vi "Power Accuracy Format Plot.vi"(6 "Calculated Values":refnum<vi>, 8 "error in (no error)":errorcluster, 9 "Reset Plot? (F)":bool, 10 "Test Parameters":T1={"Stimulus"={"Power Start"=38, "Power Stop"=46, "Frequency Type"=enum."Band Edges", "Frequency Points"=[], "TX 1 Frequency (MHz)"={"Min"=0.0, "Max"=0.0}, "TX 2 Frequency (MHz)"={"Min"=0.0, "Max"=0.0}, "RX Frequency (MHz)"={"Min"=0.0, "Max"=0.0}, "Pad Model Number"="", "Pad Serial Number"="", "Pad Values"=[]}, "Measurement"={"DUT Port"=enum."Port 1", "Direction"=0}, "Display"={"Power"={"Min"=0, "Max"=0}, "Tolerance"={"Min"=0.0, "Max"=0.0}}, "Limit"={"Tolerance"=0.35}, "Calibration"={"Calibrated?"=FALSE}} {"Measurement"."Direction" items=["Reverse", "Forward", "Auxiliary"]}, 11 "Plots":T9) -> (0 "error out":errorcluster)   [LabVIEW 2011]
uses:
  TypeDefs/Power Accuracy Test Parameters.ctl
  TypeDefs/Power Accuracy Stimulus Parameters.ctl
  TypeDefs/Power Accuracy Measurement Parameters.ctl
  SI.LIB/PIM.LIB/HW IO/DUTport.ctl
  SI.LIB/PIM.LIB/HW IO/MeasMode.ctl
  TypeDefs/Power Accuracy Display Parameters.ctl
  TypeDefs/Power Accuracy Limit Parameters.ctl
  TypeDefs/Power Accuracy Calibration State.ctl
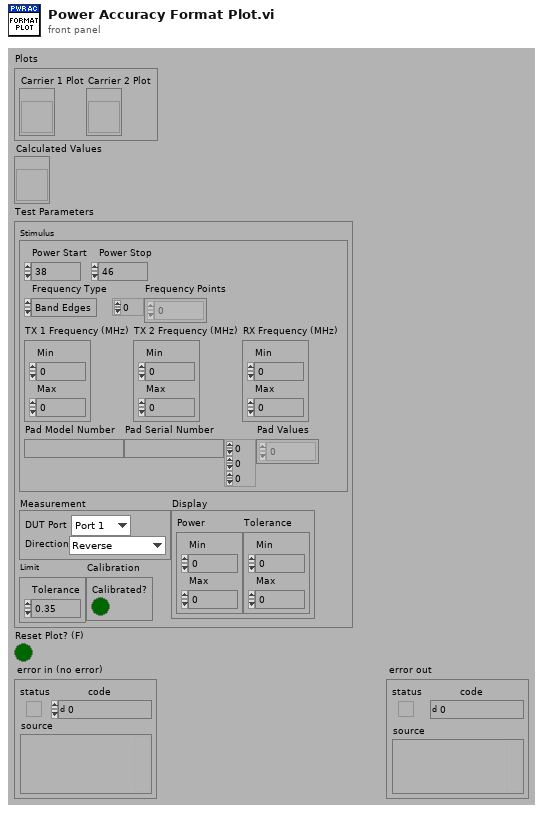
[diagram p1: front panel]
types:
  T1 = typedef "Power Accuracy Test Parameters.ctl" = cluster{"Stimulus":T2, "Measurement":T3, "Display":T6, "Limit":T7, "Calibration":T8}
  T2 = typedef "Power Accuracy Stimulus Parameters.ctl" = cluster{"Power Start":i32, "Power Stop":i32, "Frequency Type":enum16{"Band Edges", "Custom"}, "Frequency Points":dbl[], "TX 1 Frequency (MHz)":cluster{"Min":dbl, "Max":dbl}, "TX 2 Frequency (MHz)":cluster{"Min":dbl, "Max":dbl}, "RX Frequency (MHz)":cluster{"Min":dbl, "Max":dbl}, "Pad Model Number":string, "Pad Serial Number":string, "Pad Values":dbl[][][]}
  T3 = typedef "Power Accuracy Measurement Parameters.ctl" = cluster{"DUT Port":T4, "Direction":T5}
  T4 = typedef "DUTport.ctl" = enum16{"Port 1", "Port 2"}
  T5 = typedef "MeasMode.ctl" = u16
  T6 = typedef "Power Accuracy Display Parameters.ctl" = cluster{"Power":cluster{"Min":i32, "Max":i32}, "Tolerance":cluster{"Min":dbl, "Max":dbl}}
  T7 = typedef "Power Accuracy Limit Parameters.ctl" = cluster{"Tolerance":dbl}
  T8 = typedef "Power Accuracy Calibration State.ctl" = cluster{"Calibrated?":bool}
  T9 = cluster{"Carrier 1 Plot":refnum<vi>, "Carrier 2 Plot":refnum<vi>}
  T10 = cluster{"Array Constant":dbl[], "Array Constant":dbl[]}[]
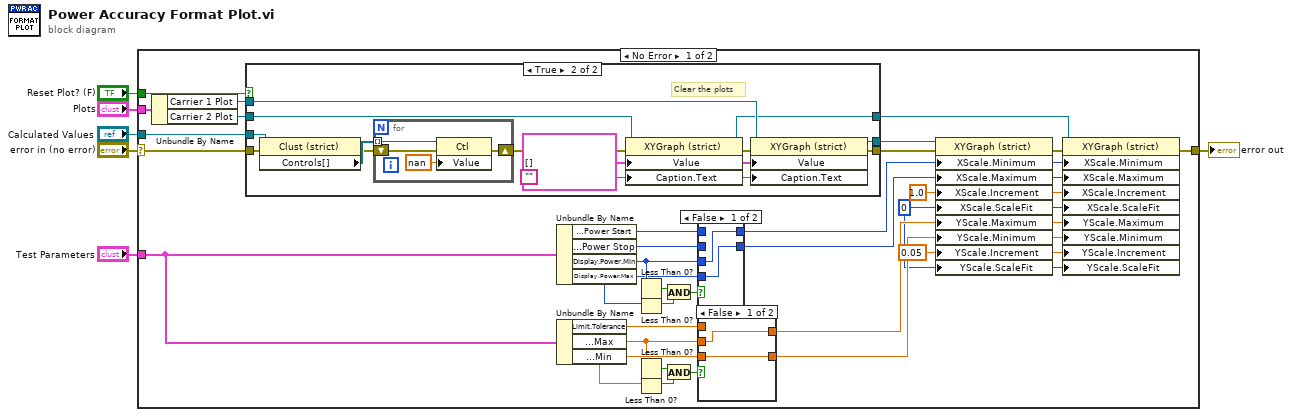
[diagram p0: block diagram]
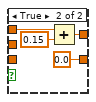
[diagram p2: hidden frame]
diagram:
  n1 = case shown="No Error" "error in (no error)" {
    selector: "error in (no error)" -> [w38 w69]
    tunnel: "Reset Plot? (F)" -> [w37 _]
    tunnel: [w15 w69] -> w5
    tunnel: "Plots" -> [w34 _]
    tunnel: "Test Parameters" -> [w18 _]
    tunnel: "Calculated Values" -> [w8 _]
    frame No Error {
      w9 = 0.05 ("Y Scale.Range:Increment")
      w7 = u8 0 ("X Scale.Scale Fit")
      w10 = 1.0 ("X Scale.Range:Increment")
      n2 = Unbundle By Name(w34) -> ("Carrier 1 Plot"=w33:refnum<vi>, "Carrier 2 Plot"=w32:refnum<vi>)
      n3 = case shown="True" w37 {
        tunnel: w38 -> [w50 w53]
        tunnel: w33 -> [w51 w64]
        tunnel: [w50 w63] -> w35
        tunnel: [w51 w62] -> w36
        tunnel: w32 -> [w49 w61]
        tunnel: [w49 w60] -> w16
        tunnel: w8 -> [_ w52]
        frame False {
        }
        frame True {
          w57 = ""
          w58 = T10 [] ("Value")
          # "Clear the plots"
          n4 = property class="Clust (strict)"(reference=w52, error in=w53) -> (error out=w55:errorcluster, "Controls[]"=w56:refnum<vi>[])  [unwired: 1 out]
          n5 = for {
            shift-right: [w67] -> w54
            shift-left: w55 -> [w68]
            tunnel: w56 -> [w66] mode=indexing
            n6 = property class="Ctl"(reference=w66, error in=w68, "Value"=nan) -> (error out=w67:errorcluster)  [unwired: 1 out]
          }
          n7 = property class="XYGraph (strict)"(reference=w61, error in=w54, "Value"=w58, "Caption.Text"=w57) -> (reference out=w60:refnum<vi>, error out=w59:errorcluster)
          n8 = property class="XYGraph (strict)"(reference=w64, error in=w59, "Value"=w58, "Caption.Text"=w57) -> (reference out=w62:refnum<vi>, error out=w63:errorcluster)
        }
      }
      n9 = Unbundle By Name(w18) -> ("Stimulus.Power Start"=w28:i32, "Stimulus.Power Stop"=w27:i32, "Display.Power.Min"=w26:i32, "Display.Power.Max"=w25:i32)
      n10 = Unbundle By Name(w18) -> ("Limit.Tolerance"=w22:dbl, "Display.Tolerance.Max"=w23:dbl, "Display.Tolerance.Min"=w24:dbl)
      n11 = Less Than 0?(x=w26) -> (x < 0?=w31:bool)
      n12 = Less Than 0?(x=w25) -> (x < 0?=w30:bool)
      n13 = Less Than 0?(x=w23) -> (x < 0?=w19:bool)
      n14 = Less Than 0?(x=w24) -> (x < 0?=w20:bool)
      n15 = And(x=w31, y=w30) -> (x .and. y?=w29:bool)
      n16 = And(x=w19, y=w20) -> (x .and. y?=w21:bool)
      n17 = case shown="False" w29 {
        tunnel: w28 -> [_ w48]
        tunnel: w27 -> [_ w47]
        tunnel: [w46 w48] -> w14
        tunnel: [w45 w47] -> w13
        tunnel: w26 -> [w46 _]
        tunnel: w25 -> [w45 _]
        frame False {
        }
        frame True {
        }
      }
      n18 = case shown="False" w21 {
        tunnel: w22 -> [_ w44]
        tunnel: [w40 w42] -> w12
        tunnel: [w39 0.0 ("Min")] -> w11
        tunnel: w23 -> [w40 _]
        tunnel: w24 -> [w39 _]
        frame False {
        }
        frame True {
          n19 = Add(x=w44, y=0.15) -> (x+y=w42:dbl)
        }
      }
      n20 = property class="XYGraph (strict)"(reference=w36, error in=w35, "XScale.Minimum"=w14, "XScale.Maximum"=w13, "XScale.Increment"=w10, "XScale.ScaleFit"=w7, "YScale.Maximum"=w12, "YScale.Minimum"=w11, "YScale.Increment"=w9, "YScale.ScaleFit"=w7) -> (error out=w17:errorcluster)  [unwired: 1 out]
      n21 = property class="XYGraph (strict)"(reference=w16, error in=w17, "XScale.Minimum"=w14, "XScale.Maximum"=w13, "XScale.Increment"=w10, "XScale.ScaleFit"=w7, "YScale.Maximum"=w12, "YScale.Minimum"=w11, "YScale.Increment"=w9, "YScale.ScaleFit"=w7) -> (error out=w15:errorcluster)  [unwired: 1 out]
    }
    frame Error {
    }
  }
  "error out" <- w5
